vi "Raise pause flag.vi"(8 "error in (no error)":errorcluster, 11 "Monkey in":refnum<class "Monkey.lvclass">) -> (0 "error out":errorcluster, 3 "Monkey out":refnum<class "Monkey.lvclass">)   [LabVIEW 2020, in "Monkey.lvlib" / "Monkey.lvclass"]
doc: "Negate the pause flag if the stopped flag wasn't raised. Show/hide indicator"
uses:
  Monkey.lvclass
  Monkey.lvclass/Monkey.ctl
  TALOS/TALOS_PPL.lvlibp/Father of all uServices/Father of all uServices/Father of all uServices.lvclass
  C:/Users/aegis/Documents/CIRCUS/TALOS/TALOS_PPL.lvlibp/Father of all uServices/Father of all uServices/Father of all uServices.lvclass
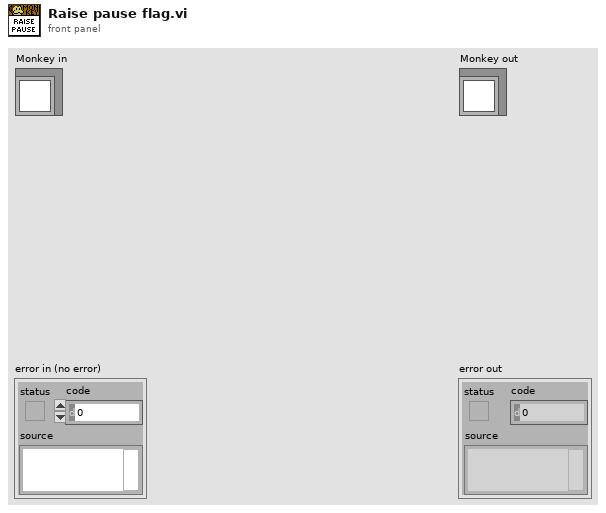
[diagram p1: front panel]
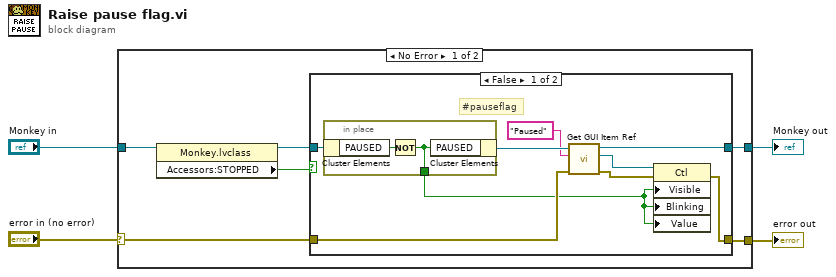
[diagram p0: block diagram]
diagram:
  n1 = case shown="No Error" "error in (no error)" {
    selector: "error in (no error)" -> [w7 w25]
    tunnel: [w9 w25] -> w3
    tunnel: [w10 w24] -> w1
    tunnel: "Monkey in" -> [w8 w24]
    frame No Error {
      n2 = property class="Monkey.lvclass"(reference=w8) -> (reference out=w6:refnum<class "Monkey.lvclass">, "Accessors:STOPPED"=w5:bool)  [unwired: 1 in, 1 out]
      n3 = case shown="False" w5 {
        tunnel: [w16 w23] -> w10
        tunnel: [w15 w22] -> w9
        tunnel: w6 -> [w12 w23]
        tunnel: w7 -> [w13 w22]
        frame False {
          # "#pauseflag"
          n4 = in-place {
            in-place-border: [w20] -> w11
            n5 = in-place-cluster #1(w12) -> ("PAUSED"=w21:bool)
            n6 = Not(x=w21) -> (.not. x?=w20:bool)
            n7 = in-place-cluster #1("PAUSED"=w20) -> (w19:refnum<class "Monkey.lvclass">)
          }
          n8 = call "Get GUI Item Ref.vi"("error in (no error)"=w13, "FP Item Name"="Paused", "uService Template in"=w19) -> ("error out"=w14:errorcluster, "Ctl Refnum"=w17:refnum<vi>, "uService Template out"=w16:refnum<class "Monkey.lvclass">)  [unwired: 6 in]
          n9 = property class="Ctl"(reference=w17, error in=w14, "Visible"=w11, "Blinking"=w11, "Value"=w11) -> (error out=w15:errorcluster)  [unwired: 1 out]
        }
        frame True {
          # "stopped, so there is nothing to pause"
        }
      }
    }
    frame Error {
    }
  }
  "error out" <- w3
  "Monkey out" <- w1
